vi "niRFUtil MEAS Mean (real array).vi"(7 "Real Array":T1 min=0 max=127 format="%.2f") -> (8 "Mean":sgl format="%.2f")   [LabVIEW 2015, in "niRFUtil.lvlib"]
doc: "(c) Copyright 2006, National Instruments, Inc. This VI may not be duplicated, sold, or distributed without written consent from National Instruments."
uses:
  niRFUtil.lvlib
  Includes/niRFUtil INC Real Array.ctl
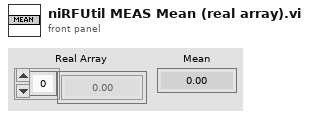
[diagram p1: front panel]
types:
  T1 = typedef "niRFUtil.lvlib/niRFUtil INC Real Array.ctl" = sgl[]
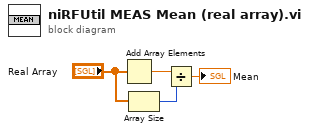
[diagram p0: block diagram]
diagram:
  n1 = Add Array Elements(numeric array="Real Array") -> (sum=w4:sgl)
  n2 = Array Size(array="Real Array") -> (size(s)=w3:i32)
  n3 = Divide(x=w4, y=w3) -> (x/y=→"Mean":sgl)
